vi "XIPIN_G.975.1_EFEC_I.7_Encoder_Decoder_2_0.vi"   [LabVIEW 2017]
doc: "The G.975.1 EFEC I.7 Encoder/Decoder LogiCore is a high speed, compact module that implements the ITU G.975.1 Enhanced Forward Error Correction with 7% overhead as specified in Annex I.7 of the standard.\n------------------------------------\n<b>Need License</b> : Yes\n<b>Interface</b> : AXI4-Stream"
uses:
  <vilib>/rvi/XilinxIP/XIPIN_XNode/niFpgaXIPIN.xnode
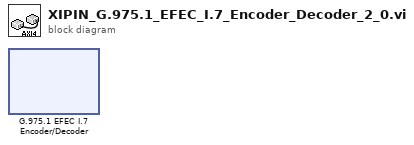
[diagram p0: block diagram]
diagram:
  n1 = xnode ("G.975.1 EFEC I.7 Encoder/Decoder")() -> ()
